vi "Alp Dev Alloc.vi"(8 "error in (no error)":errorcluster, 9 "DeviceIdPtr":u32, 10 "InitFlag":i32, 11 "DeviceNum":i32) -> (0 "error out":errorcluster, 1 "DeviceIdPtr out":u32, 3 "function return":i32)   [LabVIEW 2013, in "alpD41.lvlib"]
doc: "ALP_API long ALP_ATTR AlpDevAlloc( long DeviceNum, long InitFlag, ALP_ID* DeviceIdPtr);"
uses:
  alpD41.lvlib
  alpD41.dll
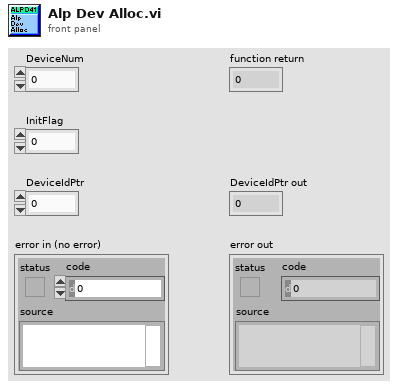
[diagram p1: front panel]
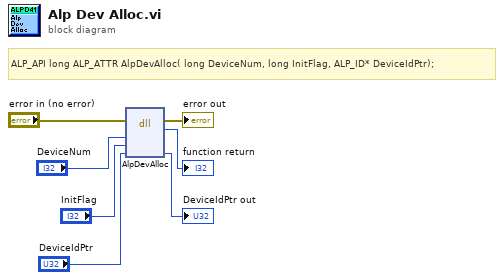
[diagram p0: block diagram]
diagram:
  # "ALP_API long ALP_ATTR AlpDevAlloc( long DeviceNum, long InitFlag, ALP_ID* DeviceIdPtr);"
  n1 = dll-call lib="C:/Users/ErNa/Google Drive (ernajqi@gmail.com)/ErNa/LabView/DMD Standalone Codes/Libraries-alpD41/alpD41.*" fn="AlpDevAlloc"(error in="error in (no error)", "DeviceNum"="DeviceNum", "InitFlag"="InitFlag", "DeviceIdPtr"="DeviceIdPtr") -> (error out=→"error out":errorcluster, →"function return":i32, "DeviceIdPtr"=→"DeviceIdPtr out":u32)  [unwired: 4 in, 1 out]
